vi "Thorlabs_SC10_Serial.vi"() -> ()   [LabVIEW 2022 SP3]
uses:
  <vilib>/Instr/_visa.llb/VISA Configure Serial Port (Instr).vi
panel:
  out "Open?":bool
  out "error out":errorcluster
  in  "error in (no error)":errorcluster
  in  "stop":bool
  in  "Open/close":bool
  in  "VISA resource name":refnum<visa-resource-name>="COM1"
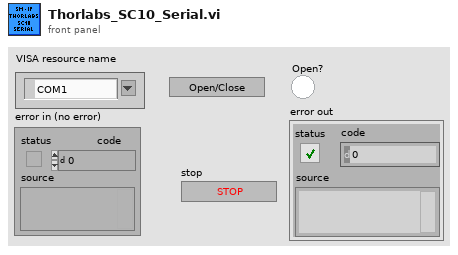
[diagram p1: front panel]
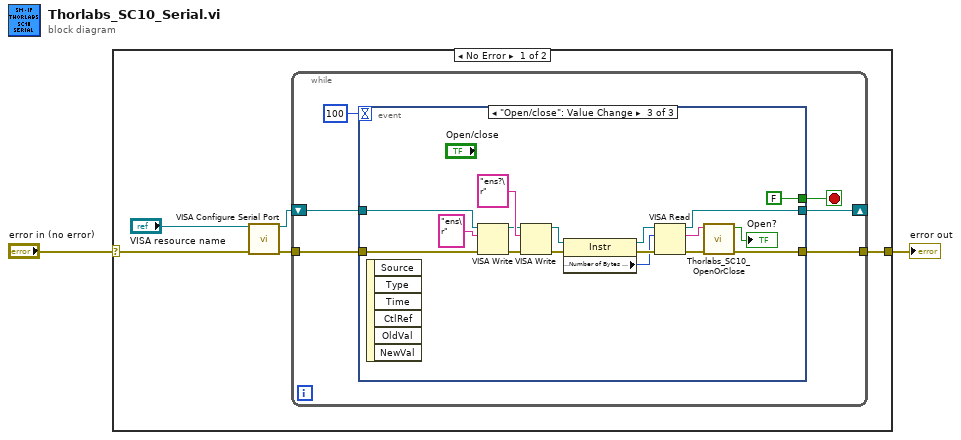
[diagram p0: block diagram]
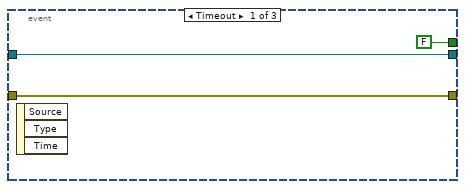
[diagram p2: hidden frame]
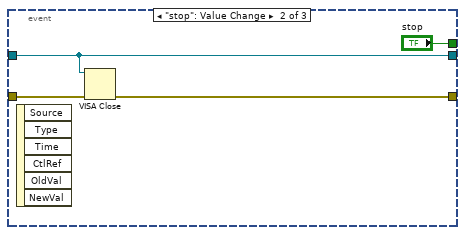
[diagram p3: hidden frame]
diagram:
  n1 = case shown="No Error" "error in (no error)" {
    selector: "error in (no error)" -> [w3 w38]
    tunnel: [w4 w38] -> w2
    frame No Error {
      n2 = call-poly "VISA Configure Serial Port"("VISA resource name"="VISA resource name", "error in (no error)"=w3) -> ("VISA resource name out"=w6:refnum<visa-resource-name>, "error out"=w5:errorcluster)  [unwired: 7 in, 5 out]
      n3 = while {
        tunnel: w5 -> [w12]
        shift-right: [w8] -> _
        shift-left: w6 -> [w11]
        tunnel: [w9] -> w4
        stop <- w10 stop-if-true
        n4 = event shown="[2] \"Open/close\": Value Change" {
          selector: _ -> [_ _ _]
          dyn-events: _ -> [_ _ _]
          timeout: 100 -> [_ _ _]
          tunnel: w12 -> [w14 w19 w36]
          tunnel: w11 -> [w15 w17 w35]
          tunnel: [w15 w17 w27] -> w8
          tunnel: [FALSE ("stop") "stop" FALSE ("stop")] -> w10
          tunnel: [w14 w18 w25] -> w9
          event Timeout {
            n5 = event-data() -> ()  [unwired: 1 in, 3 out]
          }
          event "stop": Value Change {
            n6 = event-data() -> ()  [unwired: 1 in, 6 out]
            n7 = VISA Close(VISA resource name=w17, error in (no error)=w19) -> (error out=w18:errorcluster)
          }
          event "Open/close": Value Change {
            n8 = event-data() -> ()  [unwired: 1 in, 6 out]
            n9 = VISA Write(VISA resource name=w35, write buffer="ens\r" ("Command"), error in (no error)=w36) -> (VISA resource name out=w29:refnum<visa-resource-name>, error out=w28:errorcluster)  [unwired: 1 out]
            n10 = VISA Write(VISA resource name=w29, write buffer="ens?\r" ("Command"), error in (no error)=w28) -> (VISA resource name out=w22:refnum<visa-resource-name>, error out=w21:errorcluster)  [unwired: 1 out]
            n11 = property class="Instr"(reference=w22, error in=w21) -> (reference out=w32:refnum<visa-resource-name>, error out=w31:errorcluster, "Serial Settings:Number of Bytes at Serial Port"=w30:u32)
            n12 = VISA Read(VISA resource name=w32, byte count=w30, error in (no error)=w31) -> (VISA resource name out=w27:refnum<visa-resource-name>, read buffer=w26:string, error out=w24:errorcluster)  [unwired: 1 out]
            n13 = call "Thorlabs_SC10_OpenOrClose.vi"("error in (no error)"=w24, "Input string"=w26) -> ("error out"=w25:errorcluster, "Open?"=→"Open?":bool)  [unwired: 8 in]
          }
        }
      }
    }
    frame Error {
    }
  }
  "error out" <- w2
